vi "VariantParcer.vi"(1 "Variant":variant) -> (0 "TreeItems[]":T1(array[cluster]))   [LabVIEW 2021, in "Tree.lvlib" / "Tree.lvclass"]
uses:
  Tree.lvclass
  <vilib>/Utility/Data Type/Type Definitions/Data Type.ctl
  <vilib>/Utility/Data Type/NI_Data Type.lvlib
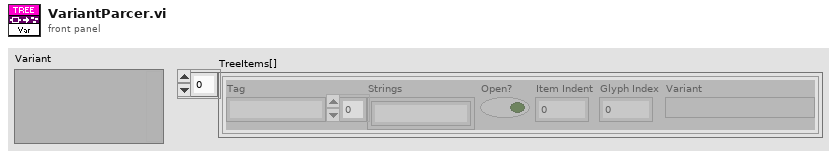
[diagram p1: front panel]
types:
  T1 = cluster{"Tag":string, "Strings":string[], "Open?":bool, "Item Indent":i32, "Glyph Index":i32, "Variant":variant}[]
  T2 = typedef "NI_Data Type.lvlib/Data Type.ctl" = enum8{"Invalid Type", "Void", "I8", "I16", "I32", "I64", "U8", "U16", "U32", "U64", "Single Float", "Double Float", "Extended Float", "Single Complex", "Double Complex", "Extended Complex", "Enum U8", "Enum U16", "Enum U32", "Enum U64", "Single Float With Unit", "Double Float With Unit", "Extended Float With Unit", "Single Complex with Unit", "Double Complex with Unit", "Extended Complex with Unit", "Boolean", "String", "Path", "Picture", "Tag", "Array", "Cluster", "Variant", "LV Variant", "Waveform", "Timestamp", "Digital Waveform", "Digital Data", "ExpressData", "Refnum", "External Data", "VI", "Poly VI", "LabVIEW Class Instance", "Fixed Point", "Set Collection", "Map Collection"}
  T3 = cluster{"Path":string, "Type":T2, "Label":string, "Value":string}[]
  T4 = cluster{"use system decimal point (T)":bool, "width (-)":i16, "precision (6)":i16}
  T5 = cluster{"Left Cell String":string, "Child Text":string[], "Child Tag":string, "Item Indent":i32, "Child Only?":bool, "Glyph Index":i32}[]
  T6 = cluster{"Tag":string, "Strings":string[], "Open?":bool, "Item Indent":i32, "Glyph Index":i32, "Variant":variant}
  T7 = cluster{"Left Cell String":string, "Child Text":string[], "Child Tag":string, "Item Indent":i32, "Child Only?":bool, "Glyph Index":i32}
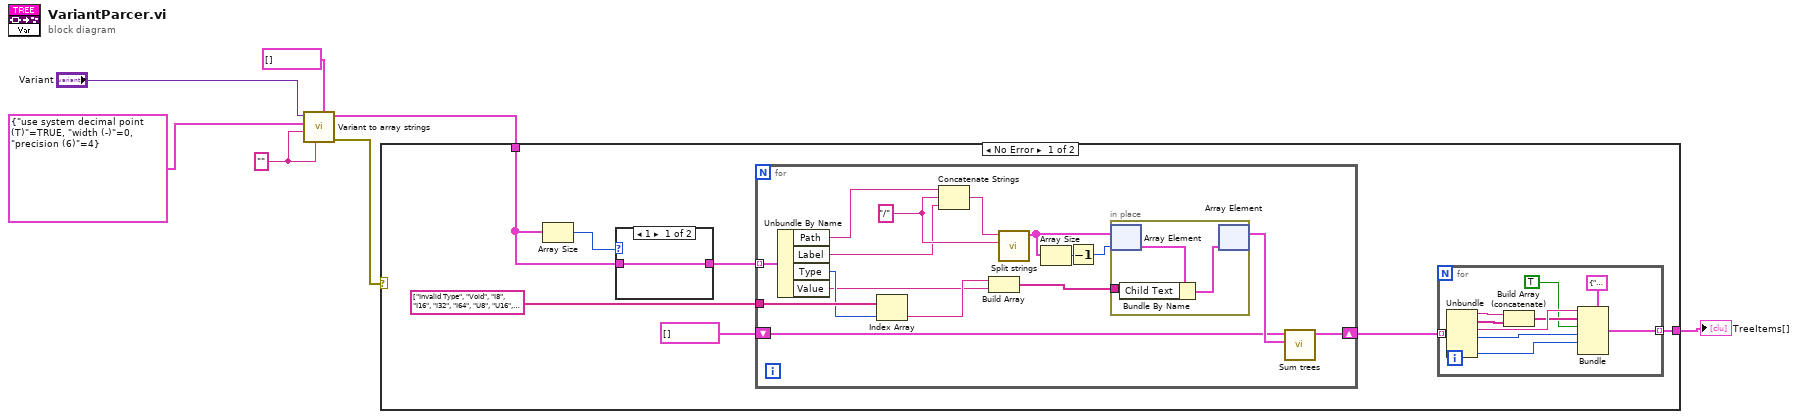
[diagram p0: block diagram]
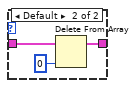
[diagram p2: hidden frame]
diagram:
  w2 = "" ("Path")
  n1 = call "Variant to array strings.vi"("cluster"=T3 [], "Array index"=w2, "Path"=w2, "Params"=T4 {"use system decimal point (T)"=TRUE, "width (-)"=0, "precision (6)"=4}, "Variant"="Variant") -> ("Error out"=w4:errorcluster, "output array"=w3:T3)  [unwired: 5 in]
  n2 = case shown="No Error" w4 {
    tunnel: w3 -> [w11 _]
    tunnel: [w8 _] -> w1
    frame No Error {
      n3 = Array Size(array=w11) -> (size(s)=w10:i32)
      n4 = case shown="1" w10 {
        tunnel: [w25 w28] -> w12
        tunnel: w11 -> [w25 w26]
        frame 1 {
        }
        frame Default {
          n5 = Delete From Array(array=w26, index=0) -> (array with subset deleted=w28:T3)  [unwired: 1 in, 1 out]
        }
      }
      n6 = for {
        tunnel: w12 -> [w44] mode=indexing
        shift-right: [w42] -> w9
        shift-left: T5 [] ("Tree out") -> [w29]
        tunnel: string[] ["Invalid Type", "Void", "I8", "I16", "I32", "I64", "U8", "U16", "U32", "U64", "Single Float", "Double Float", "Extended Float", "Single Complex", "Double Complex", "Extended Complex", "Enum U8", "Enum U16", "Enum U32", "Enum U64", "Single Float With Unit", "Double Float With Unit", "Extended Float With Unit", "Single Complex with Unit", "Double Complex with Unit", "Extended Complex with Unit", "Boolean", "String", "Path", "Picture", "Tag", "Array", "Cluster", "Variant", "LV Variant", "Waveform", "Timestamp", "Digital Waveform", "Digital Data", "ExpressData", "Refnum", "External Data", "VI", "Poly VI", "LabVIEW Class Instance", "Fixed Point"] ("Strings []") -> [w38]
        w40 = "/" ("regular expression")
        n7 = Unbundle By Name(w44) -> ("Path"=w43:string, "Label"=w39:string, "Type"=w37:T2, "Value"=w33:string)
        n8 = Index Array(array=w38, index=w37) -> (element=w34:string)
        n9 = Concatenate Strings(w43, w40, w39) -> (w41:string)
        n10 = Build Array(w34, w33) -> (w32:string[])
        n11 = call "Split strings.vi"("regular expression"=w40, "qualified name"=w41) -> ("Arr"=w36:T5)  [unwired: 9 in]
        n12 = Array Size(array=w36) -> (size(s)=w35:i32)
        n13 = Decrement(x=w35) -> (x-1=w31:i32)
        n14 = in-place {
          in-place-border: w32 -> [w45]
          n15 = in-place-array #1(w36, w31) -> (w47:T7)
          n16 = Bundle By Name(cluster=w47, "Child Text"=w45) -> (w46:T7)
          n17 = in-place-array #1(w46) -> (w30:T5)  [unwired: 1 out]
        }
        n18 = call "Sum trees.vi"("Add_to_tree"=w30, "Tree"=w29) -> ("Tree out"=w42:T5)  [unwired: 9 in]
      }
      n19 = for {
        tunnel: w9 -> [w24] mode=indexing
        tunnel: [w16] -> w8 mode=indexing
        n20 = Unbundle(w24) -> ("Left Cell String"=w21:string, "Child Text"=w20:string[], "Child Tag"=w22:string, "Item Indent"=w18:i32, "Glyph Index"=w17:i32)  [unwired: 1 out]
        n21 = Build Array (concatenate)(w21, w20) -> (w19:string[])
        n22 = Bundle(cluster=T6 {"Tag"="", "Strings"=[], "Open?"=FALSE, "Item Indent"=0, "Glyph Index"=0, "Variant"=variant} ("Cluster"), "Tag"=w22, "Strings"=w19, "Open?"=TRUE, "Item Indent"=w18, "Glyph Index"=w17) -> (w16:T6)  [unwired: 1 in]
      }
    }
    frame Error {
    }
  }
  "TreeItems[]" <- w1
